vi "Router - Latency Bmk - Interelaved Ch - Data Integrity.vi"() -> ()   [LabVIEW 2016]
uses:
  <vilib>/Utility/error.llb/DialogType.ctl
  <vilib>/pximc/Initialize Reader Session (DBL).vi
  <vilib>/pximc/Initialize Writer Session (DBL).vi
  <vilib>/pximc/Connect (DBL).vi
  <vilib>/pximc/Acquire Read Region (DBL).vi
  <vilib>/pximc/Acquire Write Region (DBL).vi
  <vilib>/pximc/nipximc.lvlib
  <resource>/objmgr/pximc.rc
panel:
  in  "Array":u64[](array[numeric])=[2, 2]
  out "Stopped?":bool=TRUE
  out "Waveform Chart 2":T1(graph)
  in  "Stop Button":bool
  in  "Node 2 Writer Interface":tag="PXI1Slot2" caption="interface"
  in  "Node 2 Writer Connection ID":u16=4
  in  "Node 2 Reader Interface":tag="PXI1Slot2" caption="interface"
  in  "Node 2 Reader Connection ID":u16=3
  in  "Node 1 Writer Interface":tag="PXI1Slot2" caption="interface"
  in  "Node 1 Writer Connection ID":u16=2
  in  "Node 1 Reader Interface":tag="PXI1Slot2" caption="interface"
  in  "Buffer Size":u64=250000 caption="buffer size"
  in  "Connection Timeout (s)":dbl=60.0 caption="timeout in seconds (-1)"
  in  "Node 1 Reader Connection ID":u16=1
  # "Node 1"
  # "Node 2"
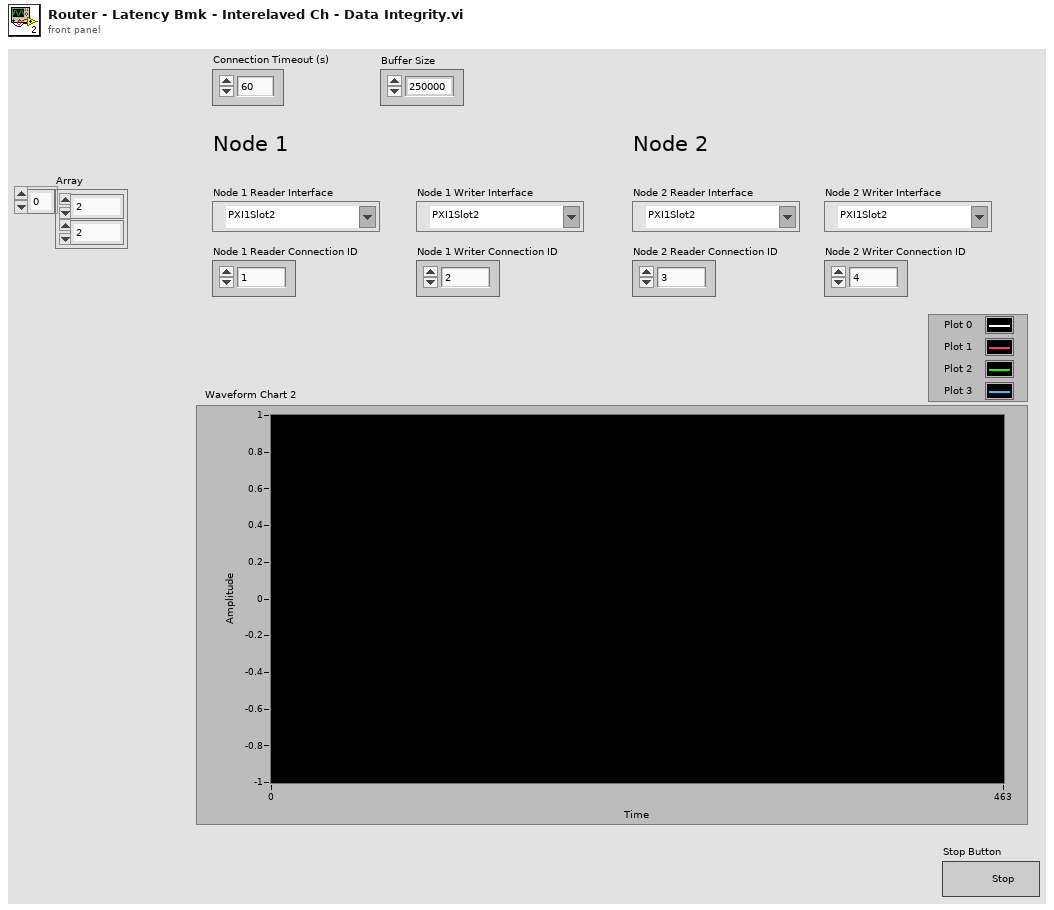
[diagram p1: front panel]
types:
  T1 = cluster{"[0]":dbl, "[1]":dbl, "[2]":dbl, "[3]":dbl, "[4]":dbl, "[5]":dbl, "[6]":dbl, "[7]":dbl, "[8]":dbl}
  T2 = typedef "DialogType.ctl" = u16
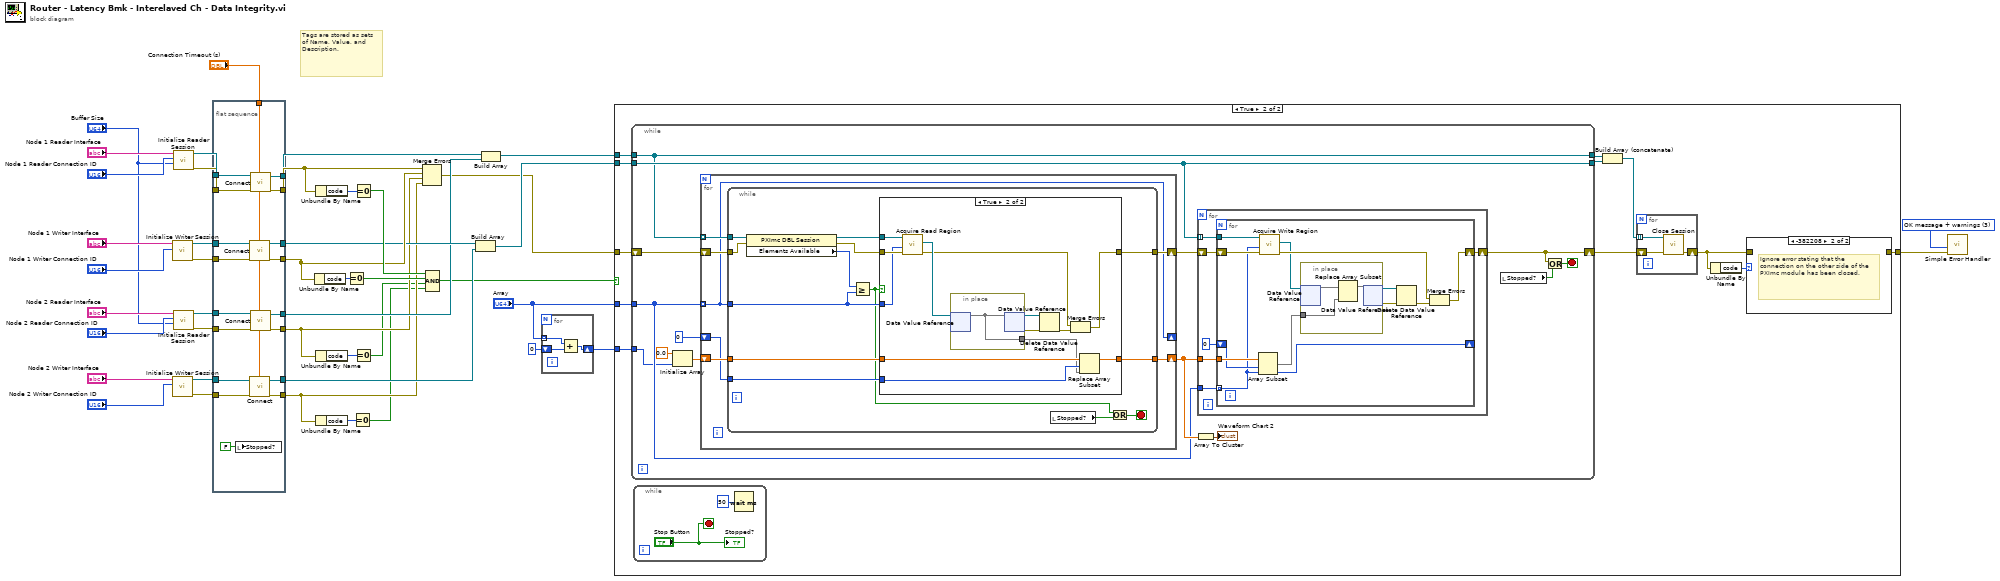
[diagram p0: block diagram]
diagram:
  w38 = T2 3 items=["no dialog", "OK message", "continue or stop message", "OK message + warnings", "continue/stop + warnings"] ("type of dialog (OK msg:1)")
  # "Tags are stored as sets of Name, Value, and Description."
  n1 = call-poly <vilib>:"Initialize Writer Session.vi"("connection id (1)"="Node 1 Writer Connection ID", "interface"="Node 1 Writer Interface") -> ("error out"=w36:errorcluster, "session out"=w35:refnum<k21>)  [unwired: 8 in]
  n2 = call-poly <vilib>:"Initialize Writer Session.vi"("connection id (1)"="Node 2 Writer Connection ID", "interface"="Node 2 Writer Interface") -> ("error out"=w24:errorcluster, "session out"=w25:refnum<k21>)  [unwired: 8 in]
  n3 = call-poly <vilib>:"Initialize Reader Session.vi"("buffer size"="Buffer Size", "writer's connection id (1)"="Node 1 Reader Connection ID", "interface"="Node 1 Reader Interface") -> ("error out"=w41:errorcluster, "session out"=w42:refnum<k21>)  [unwired: 7 in]
  n4 = call-poly <vilib>:"Initialize Reader Session.vi"("buffer size"="Buffer Size", "writer's connection id (1)"="Node 2 Reader Connection ID", "interface"="Node 2 Reader Interface") -> ("error out"=w20:errorcluster, "session out"=w19:refnum<k21>)  [unwired: 7 in]
  n5 = flat-sequence {
    tunnel: w42 -> [w61]
    tunnel: w41 -> [w60]
    tunnel: [w59] -> w15
    tunnel: w36 -> [w58]
    tunnel: w35 -> [w57]
    tunnel: [w56] -> w30
    tunnel: [w55] -> w29
    tunnel: "Connection Timeout (s)" -> [w45]
    tunnel: [w54] -> w16
    tunnel: [w53] -> w13
    tunnel: [w52] -> w11
    tunnel: [w51] -> w12
    tunnel: w25 -> [w50]
    tunnel: w24 -> [w49]
    tunnel: [w48] -> w14
    tunnel: w20 -> [w47]
    tunnel: w19 -> [w46]
    frame #0 {
      n6 = local write "Stopped?"(FALSE ("Stopped?")) -> ()
      n7 = call-poly <vilib>:"Connect.vi"("timeout in seconds (-1)"=w45, "error in (no error)"=w58, "session in"=w57) -> ("error out"=w55:errorcluster, "session out"=w54:refnum<k21>)  [unwired: 7 in]
      n8 = call-poly <vilib>:"Connect.vi"("timeout in seconds (-1)"=w45, "error in (no error)"=w49, "session in"=w50) -> ("error out"=w52:errorcluster, "session out"=w53:refnum<k21>)  [unwired: 7 in]
      n9 = call-poly <vilib>:"Connect.vi"("timeout in seconds (-1)"=w45, "error in (no error)"=w60, "session in"=w61) -> ("error out"=w56:errorcluster, "session out"=w59:refnum<k21>)  [unwired: 7 in]
      n10 = call-poly <vilib>:"Connect.vi"("timeout in seconds (-1)"=w45, "error in (no error)"=w47, "session in"=w46) -> ("error out"=w51:errorcluster, "session out"=w48:refnum<k21>)  [unwired: 7 in]
    }
  }
  n11 = Unbundle By Name(w29) -> ("code"=w33:i32)
  n12 = Unbundle By Name(w30) -> ("code"=w39:i32)
  n13 = Unbundle By Name(w12) -> ("code"=w22:i32)
  n14 = Unbundle By Name(w11) -> ("code"=w27:i32)
  n15 = Equal To 0?(x=w33) -> (x = 0?=w31:bool)
  n16 = Equal To 0?(x=w27) -> (x = 0?=w9:bool)
  n17 = Equal To 0?(x=w39) -> (x = 0?=w32:bool)
  n18 = Equal To 0?(x=w22) -> (x = 0?=w10:bool)
  n19 = Merge Errors(w30, w29, w12, w11) -> (w4:errorcluster)
  n20 = Compound Arithmetic op=AND(w32, w31, w10, w9) -> (w5:bool)
  n21 = Build Array(w16, w13) -> (w7:refnum<k21>[])
  n22 = Build Array(w15, w14) -> (w8:refnum<k21>[])
  n23 = for {
    tunnel: "Array" -> [w63] mode=indexing
    shift-right: [w62] -> w2
    shift-left: u64 0 -> [w64]
    n24 = Add(x=w63, y=w64) -> (x+y=w62:u64)
  }
  n25 = case shown="True" w5 {
    tunnel: w8 -> [_ w77]
    tunnel: w7 -> [_ w76]
    tunnel: [w65 w69] -> w6
    tunnel: w4 -> [w65 w68]
    tunnel: "Array" -> [_ w67]
    tunnel: w2 -> [_ w66]
    frame False {
    }
    frame True {
      n26 = while {
        tunnel: w77 -> [w84]
        tunnel: w76 -> [w89]
        shift-right: [w91] -> w74
        shift-left: w68 -> [w90]
        tunnel: [w84] -> w73
        tunnel: [w89] -> w72
        tunnel: w67 -> [w83]
        tunnel: w66 -> [w82]
        stop <- w92 stop-if-true
        n27 = Initialize Array(0.0 ("element"), w82) -> (w87:dbl[])
        n28 = for {
          shift-right: [w100] -> w93
          shift-left: w90 -> [w99]
          tunnel: w84 -> [w98] mode=indexing
          shift-right: [w96] -> w85
          shift-left: w87 -> [w97]
          tunnel: w83 -> [w94] mode=indexing
          shift-right: [w94] -> _
          shift-left: u64 0 ("y") -> [w95]
          n29 = while {
            tunnel: w98 -> [w112]
            tunnel: w99 -> [w109]
            tunnel: [w113] -> w100
            tunnel: w97 -> [w107]
            tunnel: [w106] -> w96
            tunnel: w94 -> [w105]
            tunnel: w95 -> [w104]
            stop <- w101 stop-if-true
            n30 = property class="PXImc DBL Session"(reference=w112, error in=w109) -> (reference out=w110:refnum<k21>, error out=w108:errorcluster, "Elements Available"=w111:u64)
            n31 = Greater Or Equal?(x=w111, y=w105) -> (x >= y?=w103:bool)
            n32 = case shown="True" w103 {
              tunnel: w108 -> [w115 w127]
              tunnel: [w115 w121] -> w113
              tunnel: w110 -> [_ w126]
              tunnel: w107 -> [w114 w120]
              tunnel: w104 -> [_ w119]
              tunnel: [w114 w117] -> w106
              tunnel: w105 -> [_ w116]
              frame False {
              }
              frame True {
                n33 = call-poly <vilib>:"Acquire Read Region.vi"("error in (no error)"=w127, "number of elements"=w116, "session in"=w126) -> ("error out"=w122:errorcluster, "read region reference"=w128:refnum<data-value>)  [unwired: 5 in, 2 out]
                n34 = in-place {
                  in-place-border: [w129] -> w118
                  n35 = in-place-dvr #1(w128) -> (w129:dbl[])  [unwired: 1 out]
                  n36 = in-place-dvr #1(w129) -> (w125:refnum<data-value>, w124:errorcluster)
                }
                n37 = Delete Data Value Reference(data value reference=w125, error in=w124) -> (error out=w123:errorcluster)  [unwired: 1 out]
                n38 = Merge Errors(w122, w123) -> (w121:errorcluster)
                n39 = Replace Array Subset(array=w120, new element=w118, index=w119) -> (w117:dbl[])
              }
            }
            n40 = local read "Stopped?"() -> (w102:bool)
            n41 = Or(x=w103, y=w102) -> (x .or. y?=w101:bool)
          }
        }
        n42 = Array To Cluster(array=w85) -> (cluster=→"Waveform Chart 2":T1)
        n43 = for {
          tunnel: w89 -> [w133] mode=indexing
          tunnel: w85 -> [w132]
          tunnel: w83 -> [w131]
          shift-right: [w134] -> w91
          shift-left: w93 -> [w135]
          n44 = for {
            tunnel: w133 -> [w147]
            shift-right: [w145] -> w134
            shift-left: w135 -> [w146]
            tunnel: w132 -> [w142]
            tunnel: w131 -> [w136] mode=indexing
            shift-right: [w136] -> _
            shift-left: u64 0 ("y") -> [w137]
            n45 = Array Subset(array=w142, index=w137, length=w136) -> (w141:dbl[])
            n46 = call-poly <vilib>:"Acquire Write Region.vi"("error in (no error)"=w146, "number of elements"=w136, "session in"=w147) -> ("error out"=w144:errorcluster, "write region reference"=w143:refnum<data-value>)  [unwired: 5 in, 2 out]
            n47 = in-place {
              in-place-border: w141 -> [w148]
              n48 = in-place-dvr #2(w143) -> (w150:dbl[])  [unwired: 1 out]
              n49 = Replace Array Subset(array=w150, new element=w148) -> (w149:dbl[])  [unwired: 1 in]
              n50 = in-place-dvr #2(w149) -> (w140:refnum<data-value>, w138:errorcluster)
            }
            n51 = Delete Data Value Reference(data value reference=w140, error in=w138) -> (error out=w139:errorcluster)  [unwired: 1 out]
            n52 = Merge Errors(w144, w139) -> (w145:errorcluster)
          }
        }
        n53 = local read "Stopped?"() -> (w81:bool)
        n54 = Or(x=w91, y=w81) -> (x .or. y?=w92:bool)
      }
      n55 = while {
        stop <- "Stop Button" stop-if-true
        n56 = Wait (ms)(milliseconds to wait=u32 50) -> ()  [unwired: 1 out]
        "Stopped?" <- "Stop Button"
      }
      n57 = Build Array (concatenate)(w73, w72) -> (w71:refnum<k21>[])
      n58 = for {
        tunnel: w71 -> [w153] mode=indexing
        shift-right: [w151] -> w70
        shift-left: w74 -> [w152]
        n59 = call <vilib>:"Close Session.vi"("error in (no error)"=w152, "session in"=w153) -> ("error out"=w151:errorcluster)  [unwired: 9 in]
      }
      n60 = Unbundle By Name(w70) -> ("code"=w75:i32)
      n61 = case shown="-382208" w75 {
        tunnel: w70 -> [w154 _]
        tunnel: [w154 _] -> w69
        frame 0, Default {
        }
        frame -382208 {
          # "Ignore error stating that the connection on the other side of the PXImc module has been closed."
        }
      }
    }
  }
  n62 = call <vilib>:"Simple Error Handler.vi"("type of dialog (OK msg:1)"=w38, "error in (no error)"=w6) -> ()  [unwired: 3 in, 5 out]
